vi "Turck Ethernet IP examples.vi"   [LabVIEW 2021]
panel:
  # "Turck  Project\nTREE\n\nKirschenhofer GmbH\n(c) 2019"
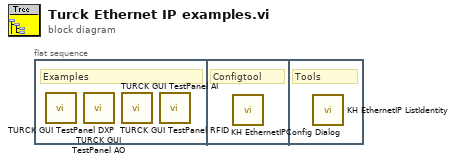
[diagram p0: block diagram]
diagram:
  n1 = flat-sequence {
    frame #0 {
      # "Examples"
      n2 = call "TURCK GUI TestPanel DXP.vi"() -> ()  [unwired: 12 in]
      n3 = call "TURCK GUI TestPanel AO.vi"() -> ()  [unwired: 12 in]
      n4 = call "TURCK GUI TestPanel AI.vi"() -> ()  [unwired: 12 in]
      n5 = call "TURCK GUI TestPanel RFID.vi"() -> ()  [unwired: 12 in]
    }
    frame #1 {
      # "Configtool"
      n6 = call "KH EthernetIPConfig Dialog.vi"() -> ()  [unwired: 10 in, 2 out]
    }
    frame #2 {
      # "Tools"
      n7 = call "KH EthernetIP ListIdentity.vi"() -> ()  [unwired: 10 in, 2 out]
    }
  }
